vi "Init.vi"(5 "EventLogger":refnum<class "EventLoggingService.lvclass">, 6 "App Version":string, 7 "SequenceCountService":refnum<class "SequenceCountService.lvclass">, 8 "error in (no error)":errorcluster, 10 "Node":refnum<class "Node Config.lvclass">) -> (0 "error out":errorcluster, 3 "DiscoveryService out":refnum<class "DiscoveryService.lvclass">)   [LabVIEW 2020, in "Vecto.lvlib" / "DiscoveryService.lvclass"]
uses:
  DiscoveryService.lvclass
  Node Config/Node Config.lvclass
  SequenceCountService/SequenceCountService.lvclass
  EventLoggingService/EventLoggingService.lvclass
  lv-volatus/messages/Discovery/Data.ctl
  lv-volatus/messages/Service/Data.ctl
  lv-volatus/messages/ServiceType/Enumeration.ctl
  DiscoveryService.lvclass/DiscoveryService.ctl
  lv-volatus/messages/ServiceType/ServiceType.lvlib
  lv-volatus/messages/Service/Service.lvlib
  lv-volatus/messages/Discovery/Discovery.lvlib
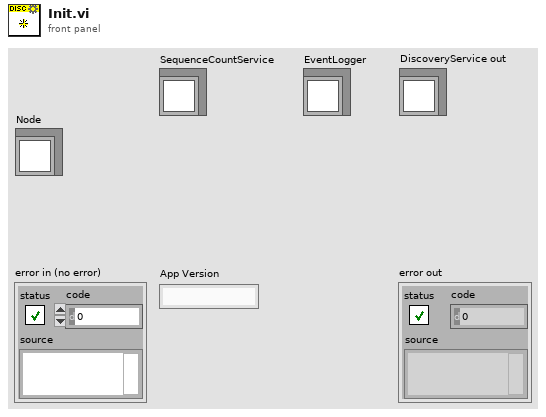
[diagram p1: front panel]
types:
  T1 = typedef "Discovery.lvlib/Data.ctl" = cluster{"node_id":u32, "name":string, "ip":u32, "status":string, "services":T2[], "capabilities":string[], "system":string, "cluster":string, "app_version":string, "cfg_version":string}
  T2 = typedef "Service.lvlib/Data.ctl" = cluster{"type":T3, "port":i32}
  T3 = typedef "ServiceType.lvlib/Enumeration.ctl" = enum16{"SERVICETYPE_UNKNOWN", "SERVICETYPE_TCPSERVER", "SERVICETYPE_HTTPSERVER"}
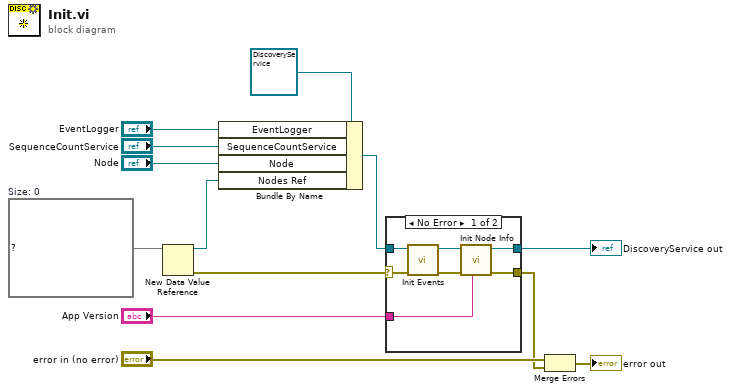
[diagram p0: block diagram]
diagram:
  w11 = map{u32, T1} {}  # Size: 0
  n1 = New Data Value Reference(data value=w11) -> (data value reference=w10:refnum<data-value>, error out=w7:errorcluster)  [unwired: 1 in]
  n2 = Bundle By Name(cluster=refnum<class "DiscoveryService.lvclass"> refnum ("DiscoveryService in"), "EventLogger"="EventLogger", "SequenceCountService"="SequenceCountService", "Node"="Node", "Nodes Ref"=w10) -> (w9:refnum<class "DiscoveryService.lvclass">)
  n3 = case shown="No Error" w7 {
    selector: w7 -> [w19 w21]
    tunnel: w9 -> [w20 w22]
    tunnel: [w15 w22] -> w8
    tunnel: [w17 w21] -> w4
    tunnel: "App Version" -> [w14 _]
    frame No Error {
      n4 = call "Init Events.vi"("error in (no error)"=w19, "DiscoveryService in"=w20) -> ("error out"=w18:errorcluster, "DiscoveryService out"=w16:refnum<class "DiscoveryService.lvclass">)  [unwired: 8 in]
      n5 = call "Init Node Info.vi"("App Version"=w14, "error in (no error)"=w18, "DiscoveryService in"=w16) -> ("error out"=w17:errorcluster, "DiscoveryService out"=w15:refnum<class "DiscoveryService.lvclass">)  [unwired: 7 in]
    }
    frame Error {
    }
  }
  "DiscoveryService out" <- w8
  n6 = Merge Errors("error in (no error)", w4) -> (→"error out":errorcluster)
